vi "Create Input Groups.vi"(8 "error in":errorcluster, 10 "Output Engine Group Names":string[](array[string]), 11 "Data Access Engine in":refnum<class "Data Access Engine.lvclass">) -> (0 "error out":errorcluster, 2 "Array":T1[](array[typedef]), 3 "Data Access Engine out":refnum<class "Data Access Engine.lvclass">)   [LabVIEW 2020, in "Modbus Master Engine.lvlib"]
uses:
  Modbus Master Engine.lvlib
  <vilib>/NI/NIVS Inline Async API/_Data Access Engine/Data Access Engine/Data Access Engine.lvclass
  <vilib>/NI/NIVS Inline Async API/_Data Access Engine/Data Access Engine/Types/Write.DVR.ctl
  <vilib>/NI/NIVS Inline Async API/_Data Access Engine/Access Type Classes/Write/Write.lvclass
  <vilib>/NI/NIVS Inline Async API/_Data Access Engine/Data Access Engine/Methods/Write.Lookup.vi
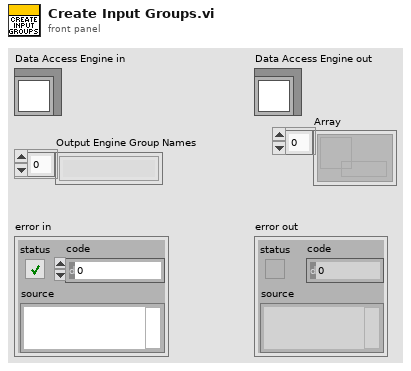
[diagram p1: front panel]
types:
  T1 = typedef "Data Access Engine.lvlib/Data Access Engine.lvclass/Write.DVR.ctl" = refnum<data-value>
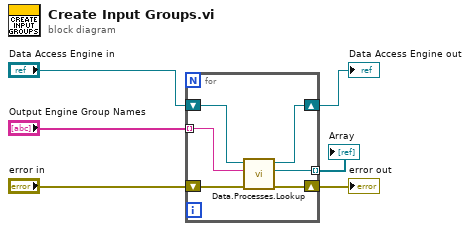
[diagram p0: block diagram]
diagram:
  n1 = for {
    tunnel: [w10] -> w1 mode=indexing
    shift-right: [w9] -> w6
    shift-left: "Data Access Engine in" -> [w12]
    shift-right: [w8] -> w3
    shift-left: "error in" -> [w11]
    tunnel: "Output Engine Group Names" -> [w7] mode=indexing
    n2 = call-poly <vilib>:"Data.Processes.Lookup.vi"("error in (no error)"=w11, "Name"=w7, "Data Access API in"=w12) -> ("error out"=w8:errorcluster, "Ref"=w10:T1, "Data Access API out"=w9:refnum<class "Data Access Engine.lvclass">)  [unwired: 5 in, 1 out]
  }
  "Data Access Engine out" <- w6
  "error out" <- w3
  "Array" <- w1
